vi "Thingworx_Write_string.vi"(9 "String":string, 11 "Thingworx":string(xcontrol)) -> ()   [LabVIEW 2020]
uses:
  TW_XControl.xctl
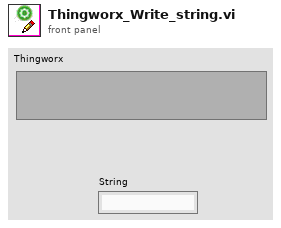
[diagram p1: front panel]
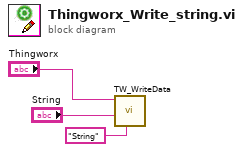
[diagram p0: block diagram]
diagram:
  n1 = call "TW_WriteData.vi"("Type"="String", "value"="String", "Property"="Thingworx") -> ()  [unwired: 9 in]
